vi "5492_SlowButton.vi"() -> ()   [LabVIEW 2017]
panel:
  in  "Dividend":dbl
  in  "Slow?":bool
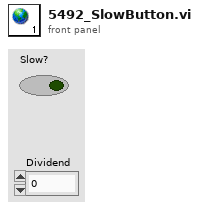
[diagram p1: front panel]
diagram:
